vi "Temperature Monitor.vi"() -> ()   [LabVIEW 2017]
doc: "This VI is the solution to an exercise in the LabVIEW Core 1 course.\n\nIt uses a While Loop and shift registers to average data. No hardware is necessary."
panel:
  in  "Stop Button":bool
  out "Temperature History":cluster{dbl, "Temperature Value":dbl}(graph)
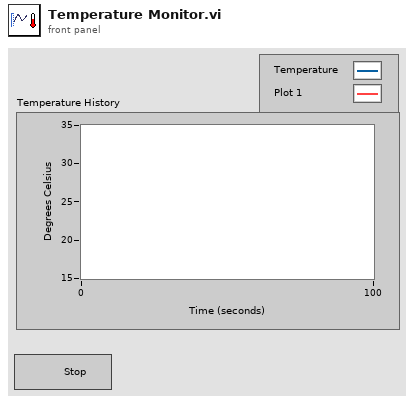
[diagram p1: front panel]
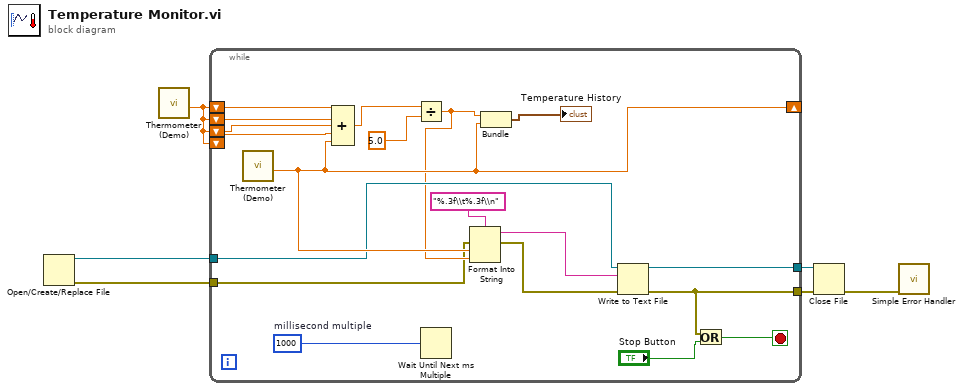
[diagram p0: block diagram]
diagram:
  n1 = Open/Create/Replace File() -> (refnum out=w2:refnum<file>, error out=w1:errorcluster)  [unwired: 6 in, 1 out]
  n2 = call "Thermometer (Demo).vi"() -> ("Temperature Value"=w6:dbl)  [unwired: 11 in]
  n3 = while {
    shift-right: [w17] -> _
    shift-left: w6 -> [w24]
    shift-left: w6 -> [w23]
    shift-left: w6 -> [w22]
    shift-left: w6 -> [w21]
    tunnel: [w13] -> w5
    tunnel: [w11] -> w4
    tunnel: w2 -> [w9]
    tunnel: w1 -> [w7]
    stop <- w12 stop-if-true
    w25 = u32 1000  # millisecond multiple
    n4 = call "Thermometer (Demo).vi"() -> ("Temperature Value"=w17:dbl)  [unwired: 11 in]
    n5 = Compound Arithmetic op=ADD(w24, w23, w22, w21, w17) -> (w20:dbl)
    n6 = Divide(x=w20, y=5.0) -> (x/y=w8:dbl)
    n7 = Wait Until Next ms Multiple(millisecond multiple=w25) -> ()  [unwired: 1 out]
    n8 = Format Into String(format string="%.3f\\t%.3f\\n", error in=w7, w17, w8) -> (resulting string=w15:string, error out=w16:errorcluster)  [unwired: 1 in]
    n9 = Bundle(w8, "Temperature Value"=w17) -> (→"Temperature History":cluster{dbl, "Temperature Value":dbl})  [unwired: 1 in]
    n10 = Write to Text File(file (use dialog)=w9, text=w15, error in=w16) -> (refnum out=w11:refnum<file>, error out=w13:errorcluster)  [unwired: 1 in, 1 out]
    n11 = Or(x=w13, y="Stop Button") -> (x .or. y?=w12:bool)
  }
  n12 = Close File(refnum=w4, error in=w5) -> (error out=w3:errorcluster)  [unwired: 1 out]
  n13 = call <vilib>:"Simple Error Handler.vi"("error in (no error)"=w3) -> ()  [unwired: 4 in, 5 out]
